vi "Move Distance in Specific Time.vi"(7 "Time Between Points (ms)":dbl, 8 "Error In":errorcluster, 9 "Time (s)":dbl, 10 "Distance (in)":dbl, 11 "Initial Snapshot":T2) -> (0 "Error Out":errorcluster, 2 "Motion Profile Portion":T1[](array[typedef]), 3 "Final Snapshot":T2)   [LabVIEW 2019, in "Motion Profile Generator.lvclass"]
uses:
  Motion Profile Generator.lvclass
  Type Defs/Motion Snapshot.ctl
  Type Defs/Motion Profile Point.ctl
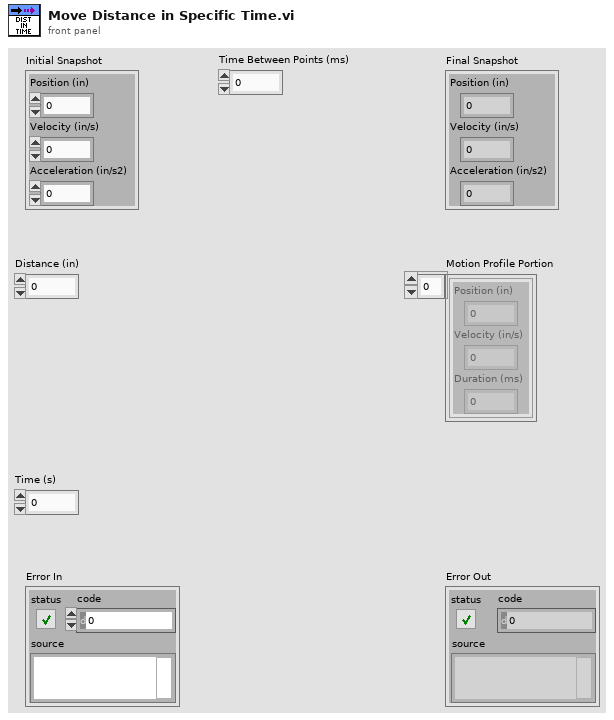
[diagram p1: front panel]
types:
  T1 = typedef "Motion Profile Generator.lvclass/Motion Profile Point.ctl" = cluster{"Position (in)":dbl, "Velocity (in/s)":dbl, "Duration (ms)":dbl}
  T2 = typedef "Motion Profile Generator.lvclass/Motion Snapshot.ctl" = cluster{"Position (in)":dbl, "Velocity (in/s)":dbl, "Acceleration (in/s2)":dbl}
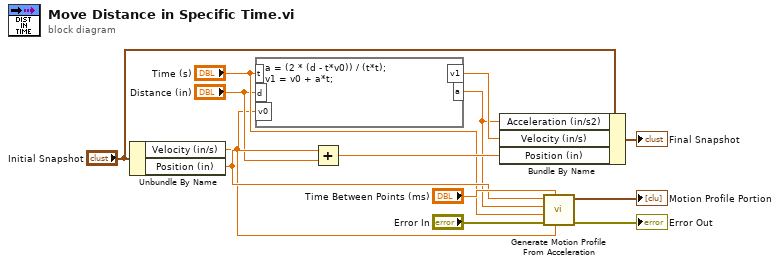
[diagram p0: block diagram]
diagram:
  n1 = Unbundle By Name("Initial Snapshot") -> ("Velocity (in/s)"=w3:dbl, "Position (in)"=w8:dbl)
  n2 = formula code="a = (2 * (d - t*v0)) / (t*t);\nv1 = v0 + a*t;"("d"="Distance (in)", "v0"=w3, "t"="Time (s)") -> ("a"=w4:dbl, "v1"=w5:dbl)
  n3 = Add(x=w8, y="Distance (in)") -> (x+y=w10:dbl)
  n4 = Bundle By Name(cluster="Initial Snapshot", "Acceleration (in/s2)"=w4, "Velocity (in/s)"=w5, "Position (in)"=w10) -> (→"Final Snapshot":T2)
  n5 = call "Generate Motion Profile From Acceleration.vi"("Initial Velocity (in/s)"=w3, "Time Between Points (ms)"="Time Between Points (ms)", "Error In"="Error In", "Movement Duration (s)"="Time (s)", "Acceleration (in/s2)"=w4, "Initial Position (in)"=w8) -> ("Error Out"=→"Error Out":errorcluster, "Motion Profile Portion"=→"Motion Profile Portion":T1[])  [unwired: 3 in, 1 out]
